vi "RunPWA_trigV2.vi"(4 "Software + buffering delay per pulse (s)":dbl=2e-06 format="%#_6e", 5 "trigger source":tag="/Dev1/PFI0", 6 "Analogue freq. (Hz)":dbl=5000.0 format="%0.2f", 7 "PW num. samples.":i32=400, 8 "PW freq. (Hz)":dbl=40.0) -> (0 "Drift of last pulse (mu. s)":dbl=-9.089951014118469e-10 format="%#_3g", 1 "Anl. / PW avg. jitter (mu.s)":dbl=212.9999999999574 format="%#_3g", 2 "Analogue data":dbl[][](array[numeric]) format="%.12f", 3 "I16 TOF (mu.s)":i16[](array[numeric])=[1380, 1279, 1463, 1254, 1163, 1317, 1629, 1097, 1100, 1774, 1172, 875, 1503, 1432, 1350, 1355, 1130, 951, 1434, 896, 1411, 1853, 1581, 1243, 1357, 886, 1545, 1268, 1475, 1942, 1228, 1498, 1306, 1554, 1663, 1181, 1453, 1038, 1198, 1321, 1316, 1534, 1316, 1839, 1620, 1542, 1789, 1374, 939, 1620, 1523, 1367, 1690, 1214, 1171, 1501, 955, 1457, 1429, 1619, 1347, 1398, 1041, 1123, 1263, 1106, 1795, 1222, 1683, 1818, 2362, 1402, 1544, 1060, 1109, 948, 1300, 1479, 1547, 1002, 1425, 1377, 2256, 1082, 1468, 2220, 1721, 1028, 1032, 1181, 1752, 1307, 1024, 1381, 1584, 1466, 1401, 902, 1473, 1422, 1798, 1715, 1444, 1316, 930, 1031, 1065, 1818, 1289, 2087, 1222, 1281, 1451, 1294, 1524, 1560, 1793, 1636, 1721, 1279, 1119, 1085, 1433, 1231, 1226, 1468, 1979, 1792, 2061, 1186, 1149, 1282, 1650, 1549, 1923, 1522, 1557, 1343, 1469, 1714, 1326, 1296, 1177, 1327, 1773, 1391, 1558, 1405, 1440, 1236, 1575, 1310, 1424, 1156, 1287, 731, 1458, 1393, 1493, 1441, 1196, 1605, 919, 1336, 1243, 1473, 1562, 1199, 1450, 1386, 1490, 1384, 1481, 1434, 1348, 1614, 1412, 1259, 2135, 1674, 1178, 1208, 1387, 1596, 1603, 1250, 1268, 1236, 1351, 1252, 1367, 1378, 1282, 1146, 1345, 1187, 1008, 1141, 1267, 1915, 1375, 1417, 1105, 1359, 1513, 1012, 1671, 1508, 1760, 1309, 1198, 1252, 1244, 1556, 1671, 1296, 1395, 1334, 1313, 1917, 1734, 1940, 1276, 1271, 1472, 1273, 981, 1430, 1391, 1038, 1236, 1167, 1419, 1935, 1188, 1658, 1317, 1217, 1663, 1432, 1498, 1494, 1620, 1528, 1200, 1603, 1200, 1514, 1288, 1327, 1644, 1311, 1573, 1033, 1669, 1022, 1624, 1999, 1993, 1489, 1519, 1483, 2032, 1397, 1345, 1706, 1229, 1299, 1063, 1269, 1192, 1609, 1377, 1299, 1538, 1347, 1231, 1262, 2060, 1816, 1442, 1713, 1096, 1593, 1807, 1549, 1242, 1353, 1506, 1533, 1551, 1097, 1770, 1588, 1253, 1313, 1345, 1658, 1527, 1551, 1780, 1001, 876, 1167, 1105, 1430, 1180, 1176, 1404, 785, 1377, 998, 1485, 1357, 952, 1304, 1477, 1138, 1303, 1281, 1376, 1603, 1495, 1690, 2050, 1558, 1238, 1430, 1341, 1126, 1070, 1743, 1649, 2205, 1470, 1632, 1677, 1210, 1669, 1968, 1267, 1394, 1582, 1865, 1256, 1582, 1356, 1535, 1791, 1637, 1226, 1787, 905, 1677, 1579, 876, 988, 1474, 1899, 1221, 1791, 1694, 1636, 1203, 1458, 1555, 1251, 1382, 954, 1185, 1240, 1264, 1228, 1298, 1885, 1489, 1702, 2401, 1725, 1110, 1190, 1572, 1369, 1223, 1131, 994, 1319, 1154, 1425, 1921, 1849, 1142, 1393, 1449, 1719, 1238, 1073, 1123, 1807, 1987])   [LabVIEW 2010]
uses:
  Kernel32.dll
  National Instruments/LabVIEW 2010/resource/objmgr/daqmx.rc
  PWAtasksGLOBAL.vi
  <vilib>/DAQmx/configure/timing.llb/DAQmx Timing (Sample Clock).vi
  <vilib>/DAQmx/configure/trigger.llb/DAQmx Start Trigger (Digital Edge).vi
  <vilib>/DAQmx/create/channels.llb/DAQmx Create Channel (DI-Digital Input).vi
  <vilib>/DAQmx/create/channels.llb/DAQmx Create Channel (DO-Digital Output).vi
  <vilib>/DAQmx/create/channels.llb/DAQmx Create Channel (AI-Voltage-Basic).vi
  <vilib>/DAQmx/read.llb/DAQmx Read (Analog 2D DBL NChan NSamp).vi
panel:
  in  "HW firing delay (s)":dbl=0.00085 format="%#_6e"
  in  "Save data?":bool
  in  "Path to save all data":path=path "C:/Documents and Settings/Aero Tunnel/Desktop/PWA vis, DAQmx and high res timer + HW/test.xls"
  in  "Analogue input channel(s)":tag="Dev1/ai0:2"
  out "PW compensated freq. (Hz)":dbl=40.003200256020484 format="%#.12g"
  in  "single shot mode for testing":bool
  out "Analogue Volts":cluster{dbl, dbl, "data":dbl[][]}(graph)={0.0, 0.0002, "data"=array3x50000[150000 elements]}
  out "PWA TOFs":cluster{"time":dbl[], i16[]}(graph)={"time"=array[400 elements], [1380, 1279, 1463, 1254, 1163, 1317, 1629, 1097, 1100, 1774, 1172, 875, 1503, 1432, 1350, 1355, 1130, 951, 1434, 896, 1411, 1853, 1581, 1243, 1357, 886, 1545, 1268, 1475, 1942, 1228, 1498, 1306, 1554, 1663, 1181, 1453, 1038, 1198, 1321, 1316, 1534, 1316, 1839, 1620, 1542, 1789, 1374, 939, 1620, 1523, 1367, 1690, 1214, 1171, 1501, 955, 1457, 1429, 1619, 1347, 1398, 1041, 1123, 1263, 1106, 1795, 1222, 1683, 1818, 2362, 1402, 1544, 1060, 1109, 948, 1300, 1479, 1547, 1002, 1425, 1377, 2256, 1082, 1468, 2220, 1721, 1028, 1032, 1181, 1752, 1307, 1024, 1381, 1584, 1466, 1401, 902, 1473, 1422, 1798, 1715, 1444, 1316, 930, 1031, 1065, 1818, 1289, 2087, 1222, 1281, 1451, 1294, 1524, 1560, 1793, 1636, 1721, 1279, 1119, 1085, 1433, 1231, 1226, 1468, 1979, 1792, 2061, 1186, 1149, 1282, 1650, 1549, 1923, 1522, 1557, 1343, 1469, 1714, 1326, 1296, 1177, 1327, 1773, 1391, 1558, 1405, 1440, 1236, 1575, 1310, 1424, 1156, 1287, 731, 1458, 1393, 1493, 1441, 1196, 1605, 919, 1336, 1243, 1473, 1562, 1199, 1450, 1386, 1490, 1384, 1481, 1434, 1348, 1614, 1412, 1259, 2135, 1674, 1178, 1208, 1387, 1596, 1603, 1250, 1268, 1236, 1351, 1252, 1367, 1378, 1282, 1146, 1345, 1187, 1008, 1141, 1267, 1915, 1375, 1417, 1105, 1359, 1513, 1012, 1671, 1508, 1760, 1309, 1198, 1252, 1244, 1556, 1671, 1296, 1395, 1334, 1313, 1917, 1734, 1940, 1276, 1271, 1472, 1273, 981, 1430, 1391, 1038, 1236, 1167, 1419, 1935, 1188, 1658, 1317, 1217, 1663, 1432, 1498, 1494, 1620, 1528, 1200, 1603, 1200, 1514, 1288, 1327, 1644, 1311, 1573, 1033, 1669, 1022, 1624, 1999, 1993, 1489, 1519, 1483, 2032, 1397, 1345, 1706, 1229, 1299, 1063, 1269, 1192, 1609, 1377, 1299, 1538, 1347, 1231, 1262, 2060, 1816, 1442, 1713, 1096, 1593, 1807, 1549, 1242, 1353, 1506, 1533, 1551, 1097, 1770, 1588, 1253, 1313, 1345, 1658, 1527, 1551, 1780, 1001, 876, 1167, 1105, 1430, 1180, 1176, 1404, 785, 1377, 998, 1485, 1357, 952, 1304, 1477, 1138, 1303, 1281, 1376, 1603, 1495, 1690, 2050, 1558, 1238, 1430, 1341, 1126, 1070, 1743, 1649, 2205, 1470, 1632, 1677, 1210, 1669, 1968, 1267, 1394, 1582, 1865, 1256, 1582, 1356, 1535, 1791, 1637, 1226, 1787, 905, 1677, 1579, 876, 988, 1474, 1899, 1221, 1791, 1694, 1636, 1203, 1458, 1555, 1251, 1382, 954, 1185, 1240, 1264, 1228, 1298, 1885, 1489, 1702, 2401, 1725, 1110, 1190, 1572, 1369, 1223, 1131, 994, 1319, 1154, 1425, 1921, 1849, 1142, 1393, 1449, 1719, 1238, 1073, 1123, 1807, 1987]}
  out "N samp. anl.":i32=50000
  out "Sampling time (s)":dbl=10.0
  out "TotalSampPerChanAcquired":dbl=50000.0
  out "AvailSampPerChan":u32
  out "CurrReadPos":dbl=50000.0
  out "Clock period (ns)":dbl=0.33336778133740486
  out "PW act. N. samps.":i32=400
  out "PW nominal dt (s)":dbl=0.025
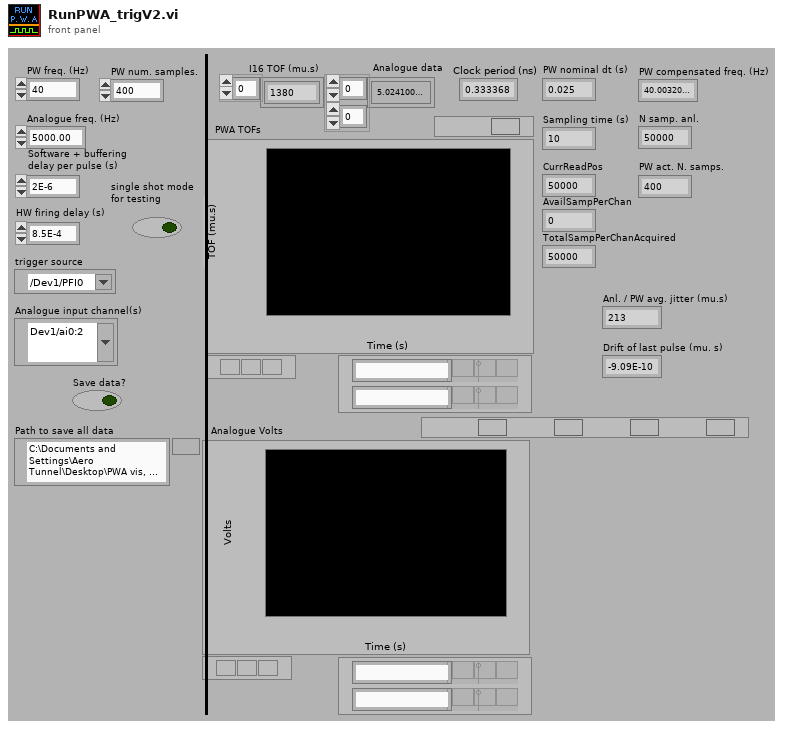
[diagram p1: front panel]
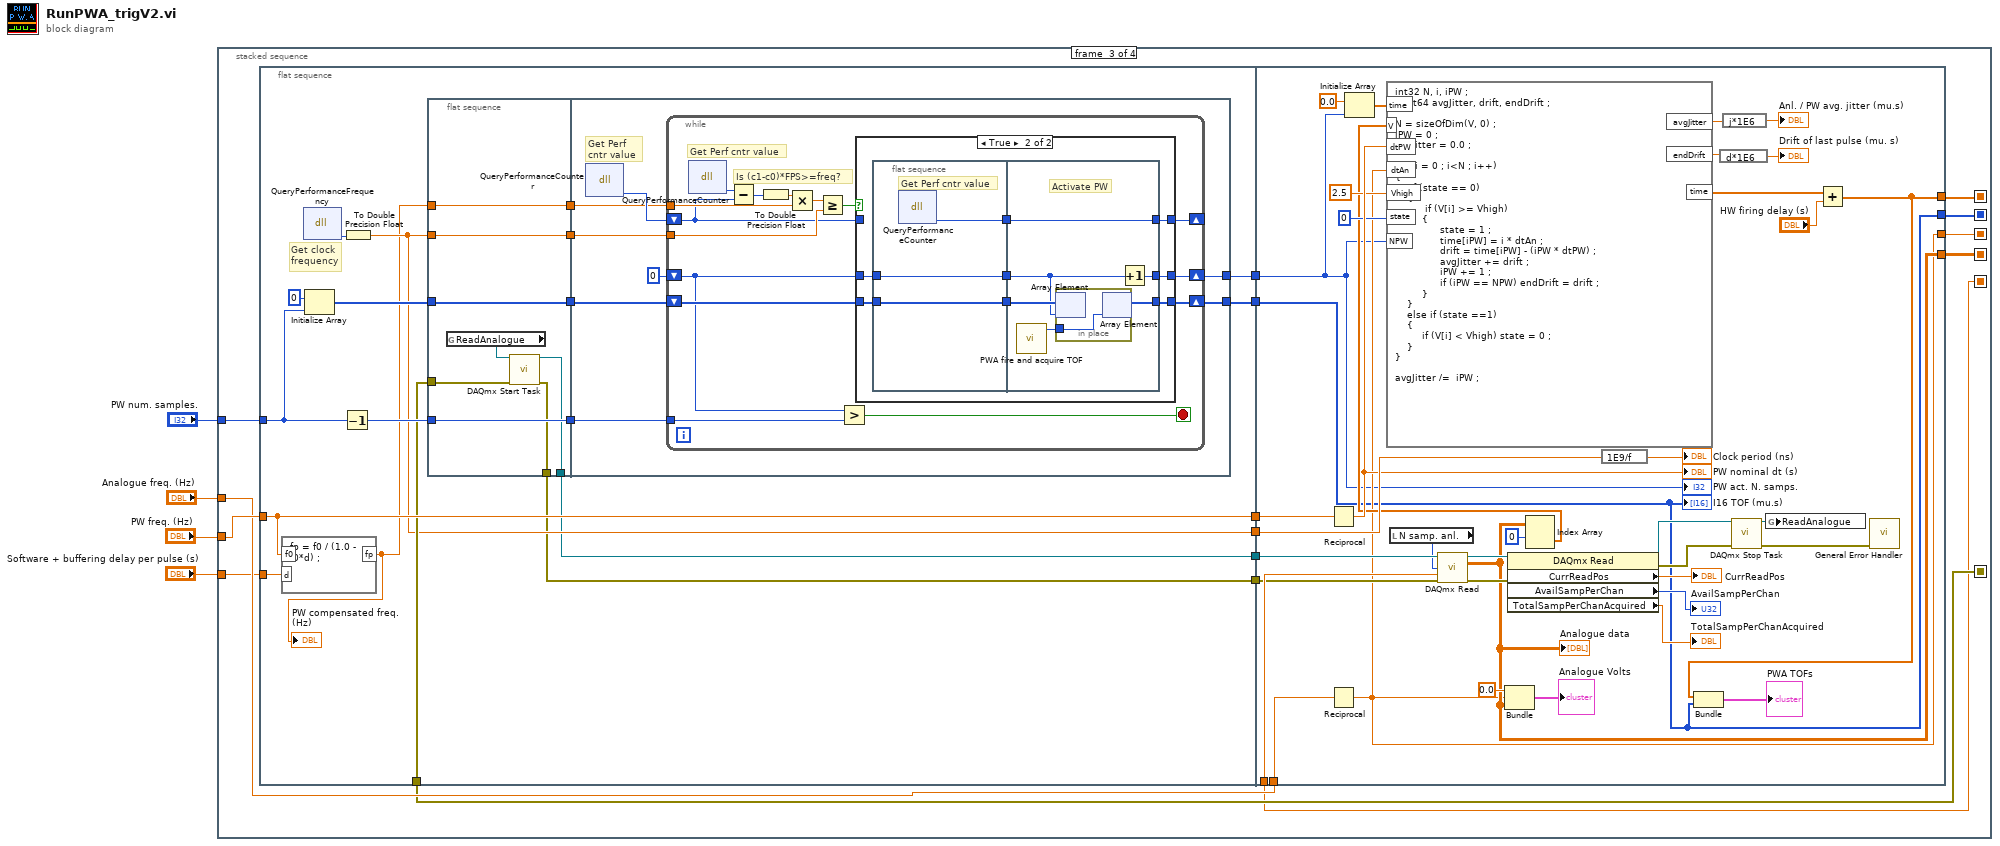
[diagram p0: block diagram]
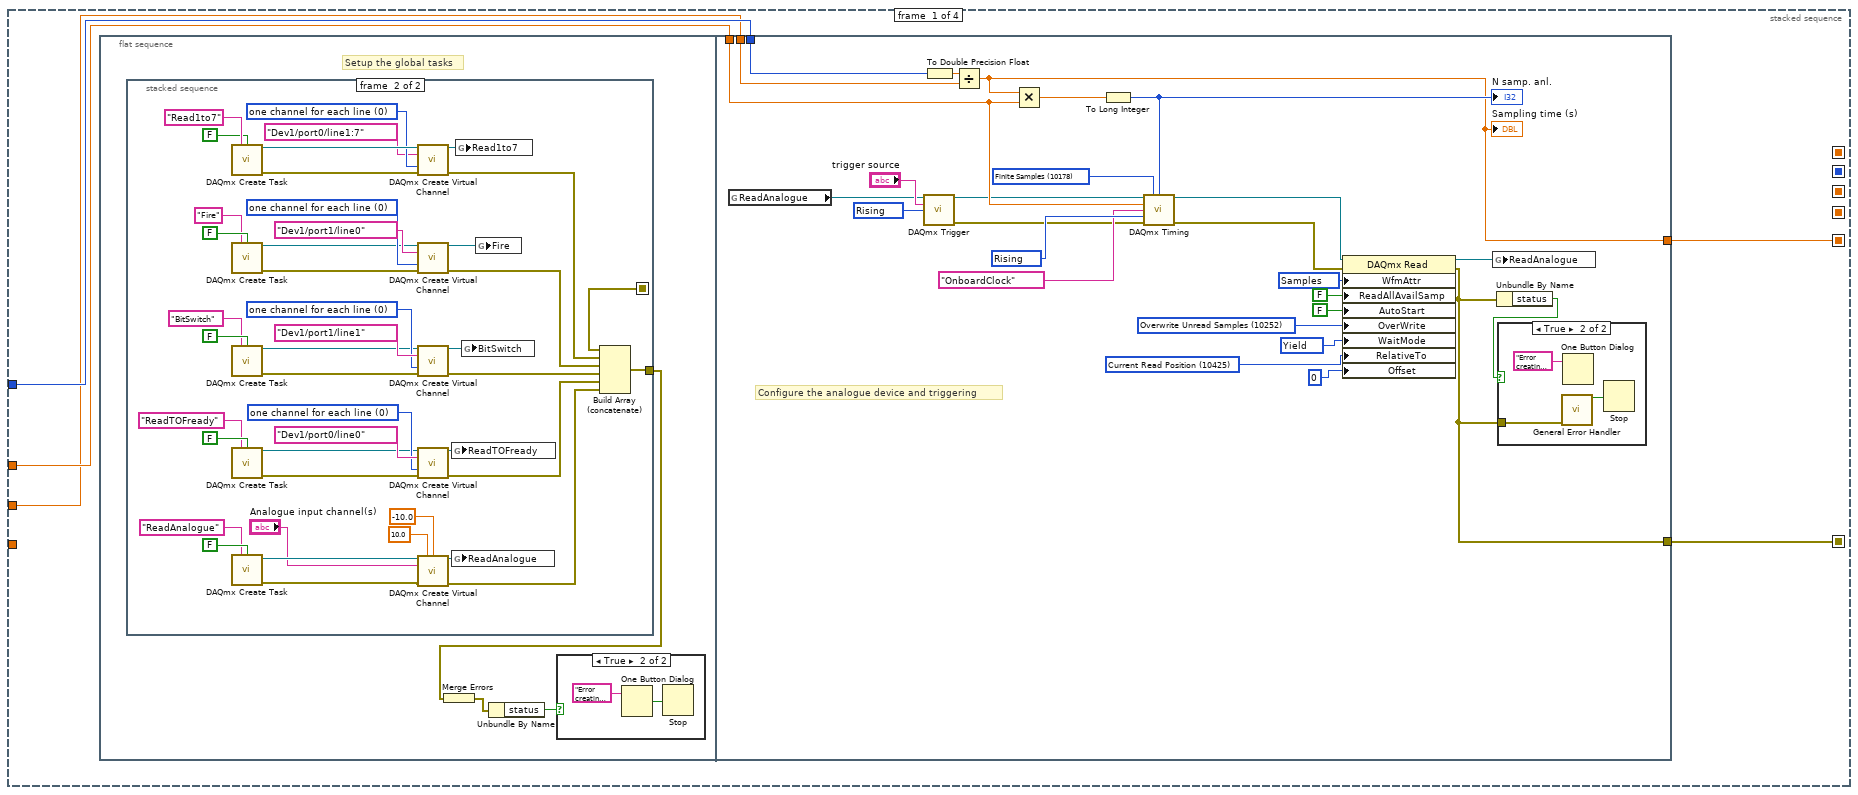
[diagram p2: hidden frame]
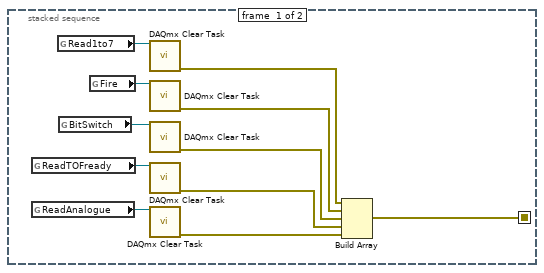
[diagram p3: hidden frame]
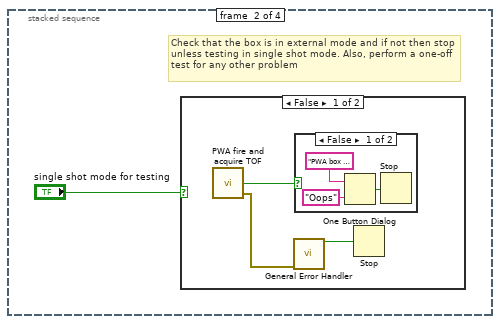
[diagram p6: hidden frame]
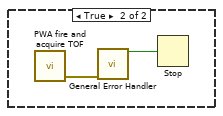
[diagram p8: hidden frame]
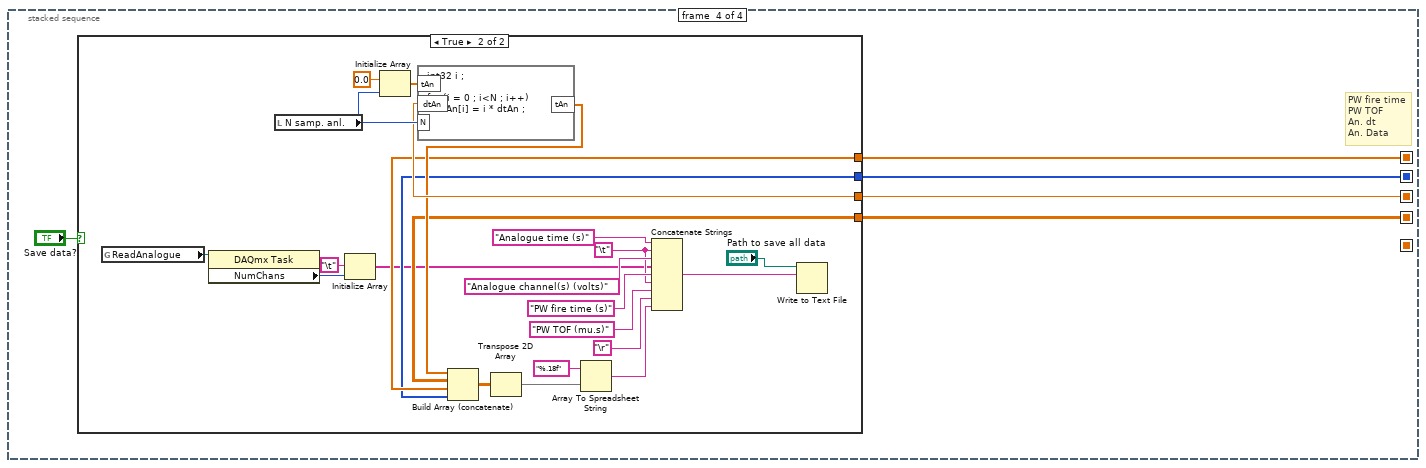
[diagram p10: hidden frame]
diagram:
  n1 = stacked-sequence {
    seq-local: [w8 _ _ _] -> [_ _ w115 _]
    seq-local: [w5 _ _ _] -> [_ _ w113 _]
    seq-local: [_ _ w111 _] -> [_ _ _ w234]
    seq-local: [_ _ w110 _] -> [_ _ _ w235]
    seq-local: [_ _ w109 _] -> [_ _ _ w236]
    seq-local: [_ _ w108 _] -> [_ _ _ w233]
    tunnel: "Analogue freq. (Hz)" -> [w9 _ w119 _]
    tunnel: "PW freq. (Hz)" -> [w6 _ w121 _]
    tunnel: "PW num. samples." -> [w7 _ w120 _]
    tunnel: "Software + buffering delay per pulse (s)" -> [_ _ w114 _]
    frame #0 {
      n2 = flat-sequence {
        tunnel: w9 -> [w81]
        tunnel: [w74] -> w8
        tunnel: w7 -> [w71]
        tunnel: w6 -> [w70]
        tunnel: [w69] -> w5
        frame #0 {
          # "Setup the global tasks"
          n3 = stacked-sequence {
            seq-local: [w13 _] -> [_ w30]
            tunnel: [_ w24] -> w11
            frame #0 {
              n4 = global read "PWAtasksGLOBAL.vi" "ReadTOFready"() -> (w20:refnum<k21>)
              n5 = global read "PWAtasksGLOBAL.vi" "ReadAnalogue"() -> (w19:refnum<k21>)
              n6 = global read "PWAtasksGLOBAL.vi" "Read1to7"() -> (w23:refnum<k21>)
              n7 = global read "PWAtasksGLOBAL.vi" "BitSwitch"() -> (w21:refnum<k21>)
              n8 = global read "PWAtasksGLOBAL.vi" "Fire"() -> (w22:refnum<k21>)
              n9 = call <vilib>:"DAQmx Clear Task.vi"("task in"=w23) -> ("error out"=w18:errorcluster)  [unwired: 14 in]
              n10 = call <vilib>:"DAQmx Clear Task.vi"("task in"=w22) -> ("error out"=w17:errorcluster)  [unwired: 14 in]
              n11 = call <vilib>:"DAQmx Clear Task.vi"("task in"=w21) -> ("error out"=w16:errorcluster)  [unwired: 14 in]
              n12 = call <vilib>:"DAQmx Clear Task.vi"("task in"=w20) -> ("error out"=w15:errorcluster)  [unwired: 14 in]
              n13 = call <vilib>:"DAQmx Clear Task.vi"("task in"=w19) -> ("error out"=w14:errorcluster)  [unwired: 14 in]
              n14 = Build Array(w18, w17, w16, w15, w14) -> (w13:errorcluster[])
            }
            frame #1 {
              w44 = 0 items=["one channel for each line", "one channel for all lines"] ("line grouping")
              w51 = 0 items=["one channel for each line", "one channel for all lines"] ("line grouping")
              w58 = 0 items=["one channel for each line", "one channel for all lines"] ("line grouping")
              w63 = 0 items=["one channel for each line", "one channel for all lines"] ("line grouping")
              n15 = call <vilib>:"DAQmx Create Task.vi"("new task name"="Read1to7", "auto cleanup"=FALSE) -> ("task out"=w64:refnum<k21>, "error out"=w60:errorcluster)  [unwired: 12 in]
              n16 = call <vilib>:"DAQmx Create Task.vi"("new task name"="Fire", "auto cleanup"=FALSE) -> ("task out"=w57:refnum<k21>, "error out"=w53:errorcluster)  [unwired: 12 in]
              n17 = call <vilib>:"DAQmx Create Task.vi"("new task name"="BitSwitch", "auto cleanup"=FALSE) -> ("task out"=w50:refnum<k21>, "error out"=w46:errorcluster)  [unwired: 12 in]
              n18 = call <vilib>:"DAQmx Create Task.vi"("new task name"="ReadTOFready", "auto cleanup"=FALSE) -> ("task out"=w43:refnum<k21>, "error out"=w39:errorcluster)  [unwired: 12 in]
              n19 = call <vilib>:"DAQmx Create Task.vi"("new task name"="ReadAnalogue", "auto cleanup"=FALSE) -> ("task out"=w38:refnum<k21>, "error out"=w34:errorcluster)  [unwired: 12 in]
              n20 = call-poly <vilib>:"DAQmx Create Virtual Channel.vi"("task in"=w64, "lines"=tag "Dev1/port0/line1:7", "line grouping"=w63, "error in"=w60) -> ("task out"=w61:refnum<k21>, "error out"=w29:errorcluster)  [unwired: 10 in]
              n21 = call-poly <vilib>:"DAQmx Create Virtual Channel.vi"("task in"=w57, "lines"=tag "Dev1/port1/line0", "line grouping"=w58, "error in"=w53) -> ("task out"=w54:refnum<k21>, "error out"=w28:errorcluster)  [unwired: 10 in]
              n22 = call-poly <vilib>:"DAQmx Create Virtual Channel.vi"("task in"=w50, "lines"=tag "Dev1/port1/line1", "line grouping"=w51, "error in"=w46) -> ("task out"=w47:refnum<k21>, "error out"=w27:errorcluster)  [unwired: 10 in]
              n23 = call-poly <vilib>:"DAQmx Create Virtual Channel.vi"("task in"=w43, "lines"=tag "Dev1/port0/line0", "line grouping"=w44, "error in"=w39) -> ("task out"=w40:refnum<k21>, "error out"=w26:errorcluster)  [unwired: 10 in]
              n24 = call-poly <vilib>:"DAQmx Create Virtual Channel.vi"("task in"=w38, "maximum value"=10.0, "minimum value"=-10.0, "physical channels"="Analogue input channel(s)", "error in"=w34) -> ("task out"=w35:refnum<k21>, "error out"=w25:errorcluster)  [unwired: 9 in]
              n25 = global write "PWAtasksGLOBAL.vi" "ReadTOFready"(w40) -> ()
              n26 = global write "PWAtasksGLOBAL.vi" "ReadAnalogue"(w35) -> ()
              n27 = global write "PWAtasksGLOBAL.vi" "Read1to7"(w61) -> ()
              n28 = global write "PWAtasksGLOBAL.vi" "BitSwitch"(w47) -> ()
              n29 = global write "PWAtasksGLOBAL.vi" "Fire"(w54) -> ()
              n30 = Build Array (concatenate)(w30, w29, w28, w27, w26, w25) -> (w24:errorcluster[])
            }
          }
          n31 = Merge Errors(w11) -> (w12:errorcluster)
          n32 = Unbundle By Name(w12) -> ("status"=w10:bool)
          n33 = case shown="True" w10 {
            frame False {
            }
            frame True {
              n34 = One Button Dialog(message="Error creating tasks, aborting") -> (true=w67:bool)  [unwired: 1 in]
              n35 = Stop(stop? (T)=w67) -> ()
            }
          }
        }
        frame #1 {
          w78 = 10280 items=["Rising"=10280, "Falling"=10171] ("edge")
          w87 = 10425 items=["First Sample"=10424, "Current Read Position"=10425, "Reference Trigger"=10426, "First Pretrigger Sample"=10427, "Most Recent Sample"=10428] ("RelativeTo")
          w88 = 12525 items=["Wait For Interrupt"=12523, "Poll"=12524, "Yield"=12525, "Sleep"=12547] ("WaitMode")
          w89 = 10252 items=["Overwrite Unread Samples"=10252, "Do Not Overwrite Unread Samples"=10159] ("OverWrite")
          w91 = 10287 items=["Samples"=10287, "Samples and Timing"=10140, "Samples, Timing, and Attributes"=10141] ("WfmAttr")
          w94 = 10280 items=["Rising"=10280, "Falling"=10171] ("active edge")
          w95 = 10178 items=["Finite Samples"=10178, "Continuous Samples"=10123, "Hardware Timed Single Point"=12522] ("sample mode")
          # "Configure the analogue device and triggering"
          n36 = global read "PWAtasksGLOBAL.vi" "ReadAnalogue"() -> (w73:refnum<k21>)
          n37 = call-poly <vilib>:"DAQmx Trigger.vi"("task/channels in"=w73, "source"="trigger source", "edge"=w78) -> ("task out"=w77:refnum<k21>, "error out"=w80:errorcluster)  [unwired: 11 in]
          n38 = To Double Precision Float(number=w71) -> (double precision float=w72:dbl)
          n39 = Divide(x=w72, y=w70) -> (x/y=w69:dbl)
          "Sampling time (s)" <- w69
          n40 = Multiply(x=w69, y=w81) -> (x*y=w83:dbl)
          n41 = To Long Integer(number=w83) -> (32bit integer=w82:i32)
          "N samp. anl." <- w82
          n42 = call-poly <vilib>:"DAQmx Timing.vi"("task/channels in"=w77, "sample mode"=w95, "samples per channel"=w82, "rate"=w81, "source"=tag "OnboardClock", "active edge"=w94, "error in"=w80) -> ("task out"=w76:refnum<k21>, "error out"=w85:errorcluster)  [unwired: 7 in]
          n43 = property class="DAQmx Read"(reference=w76, error in=w85, "WfmAttr"=w91, "ReadAllAvailSamp"=FALSE, "AutoStart"=FALSE, "OverWrite"=w89, "WaitMode"=w88, "RelativeTo"=w87, "Offset"=0) -> (reference out=w75:refnum<k21>, error out=w74:errorcluster)
          n44 = global write "PWAtasksGLOBAL.vi" "ReadAnalogue"(w75) -> ()
          n45 = Unbundle By Name(w74) -> ("status"=w84:bool)
          n46 = case shown="True" w84 {
            tunnel: w74 -> [_ w97]
            frame False {
            }
            frame True {
              n47 = call <vilib>:"General Error Handler.vi"("error in (no error)"=w97) -> ("error?"=w96:bool)  [unwired: 10 in, 4 out]
              n48 = One Button Dialog(message="Error creating tasks, aborting") -> ()  [unwired: 1 in, 1 out]
              n49 = Stop(stop? (T)=w96) -> ()
            }
          }
        }
      }
    }
    frame #1 {
      # "Check that the box is in external mode and if not then stop unless testing in single shot mode. Also, perform a one-off test for any other problem"
      n50 = case shown="False" "single shot mode for testing" {
        frame False {
          n51 = call "PWA fire and acquire TOF.vi"() -> ("Cumulative Error"=w100:errorcluster, "External mode"=w102:bool)  [unwired: 1 out]
          n52 = call <vilib>:"General Error Handler.vi"("error in (no error)"=w100) -> ("error?"=w101:bool)  [unwired: 10 in, 4 out]
          n53 = case shown="False" w102 {
            frame False {
              n54 = One Button Dialog(message="PWA box is not in external trigger mode!", button name ("OK")="Oops") -> (true=w103:bool)
              n55 = Stop(stop? (T)=w103) -> ()
            }
            frame True {
            }
          }
          n56 = Stop(stop? (T)=w101) -> ()
        }
        frame True {
          n57 = call "PWA fire and acquire TOF.vi"() -> ("Cumulative Error"=w107:errorcluster)  [unwired: 2 out]
          n58 = call <vilib>:"General Error Handler.vi"("error in (no error)"=w107) -> ("error?"=w106:bool)  [unwired: 10 in, 4 out]
          n59 = Stop(stop? (T)=w106) -> ()
        }
      }
    }
    frame #2 {
      n60 = flat-sequence {
        tunnel: [w132] -> w123
        tunnel: [w140] -> w122
        tunnel: [w139] -> w118
        tunnel: [w138] -> w117
        tunnel: [w124] -> w116
        tunnel: w115 -> [w137]
        tunnel: [w125] -> w112
        tunnel: w114 -> [w126]
        tunnel: w120 -> [w127]
        tunnel: w121 -> [w138]
        tunnel: w123 -> [w216]
        tunnel: w122 -> [w199]
        tunnel: w119 -> [w224]
        tunnel: w113 -> [w219]
        tunnel: w118 -> [w198]
        tunnel: w117 -> [w215]
        tunnel: w116 -> [w218]
        tunnel: w112 -> [w217]
        tunnel: [w195] -> w111
        tunnel: [w202] -> w110
        tunnel: [w201] -> w109
        tunnel: [w199] -> w108
        frame #0 {
          # "Get clock frequency"
          n61 = formula code="fp = f0 / (1.0 - f0*d) ;"("f0"=w138, "d"=w126) -> ("fp"=w130:dbl)
          "PW compensated freq. (Hz)" <- w130
          n62 = dll-call lib="Kernel32.dll" fn="QueryPerformanceFrequency"() -> ("Frequency"=w129:u64)  [unwired: 5 in, 2 out]
          n63 = Initialize Array(i16 0 ("Base 10 TOF (signed, \nmu.sec)"), w127) -> (w134:i16[])
          n64 = Decrement(x=w127) -> (x-1=w141:i32)
          n65 = To Double Precision Float(number=w129) -> (double precision float=w132:dbl)
          n66 = flat-sequence {
            tunnel: w137 -> [w147]
            tunnel: w141 -> [w149]
            tunnel: [w149] -> w136
            tunnel: [w146] -> w135
            tunnel: w134 -> [w146]
            tunnel: [w145] -> w133
            tunnel: w132 -> [w145]
            tunnel: [w144] -> w131
            tunnel: w130 -> [w144]
            tunnel: [w143] -> w125
            tunnel: [w142] -> w124
            tunnel: [w155] -> w140
            tunnel: [w153] -> w139
            tunnel: w136 -> [w156]
            tunnel: w135 -> [w152]
            tunnel: w133 -> [w151]
            tunnel: w131 -> [w150]
            frame #0 {
              n67 = global read "PWAtasksGLOBAL.vi" "ReadAnalogue"() -> (w148:refnum<k21>)
              n68 = call <vilib>:"DAQmx Start Task.vi"("task/channels in"=w148, "error in"=w147) -> ("task out"=w142:refnum<k21>, "error out"=w143:errorcluster)  [unwired: 12 in]
            }
            frame #1 {
              # "Get Perf cntr value"
              n69 = dll-call lib="Kernel32.dll" fn="QueryPerformanceCounter"() -> ("Counter value"=w154:u64)  [unwired: 5 in, 2 out]
              n70 = while {
                tunnel: w156 -> [w165]
                shift-right: [w172] -> _
                shift-left: w154 -> [w169]
                tunnel: w150 -> [w171]
                tunnel: w151 -> [w170]
                shift-right: [w168] -> w153
                shift-left: 0 ("Counter value") -> [w164]
                shift-right: [w167] -> w155
                shift-left: w152 -> [w166]
                stop <- w158 stop-if-true
                # "Is (c1-c0)*FPS>=freq?"
                # "Get Perf cntr value"
                n71 = dll-call lib="Kernel32.dll" fn="QueryPerformanceCounter"() -> ("Counter value"=w163:u64)  [unwired: 5 in, 2 out]
                n72 = Subtract(x=w163, y=w169) -> (x-y=w159:u64)
                n73 = To Double Precision Float(number=w159) -> (double precision float=w162:dbl)
                n74 = Multiply(x=w162, y=w171) -> (x*y=w160:dbl)
                n75 = Greater Or Equal?(x=w160, y=w170) -> (x >= y?=w161:bool)
                n76 = Greater?(x=w164, y=w165) -> (0:w158:bool)
                n77 = case shown="True" w161 {
                  tunnel: [w175 w183] -> w172
                  tunnel: w169 -> [w175 _]
                  tunnel: [w174 w182] -> w168
                  tunnel: w164 -> [w174 w181]
                  tunnel: [w173 w180] -> w167
                  tunnel: w166 -> [w173 w179]
                  frame False {
                    # "Continue looping\nuntil required time\nhas elapsed"
                  }
                  frame True {
                    n78 = flat-sequence {
                      tunnel: [w186] -> w178
                      tunnel: w181 -> [w185]
                      tunnel: [w185] -> w177
                      tunnel: w179 -> [w184]
                      tunnel: [w184] -> w176
                      tunnel: [w187] -> w183
                      tunnel: w178 -> [w187]
                      tunnel: [w192] -> w182
                      tunnel: w177 -> [w190]
                      tunnel: [w188] -> w180
                      tunnel: w176 -> [w191]
                      frame #0 {
                        # "Get Perf cntr value"
                        n79 = dll-call lib="Kernel32.dll" fn="QueryPerformanceCounter"() -> ("Counter value"=w186:u64)  [unwired: 5 in, 2 out]
                      }
                      frame #1 {
                        # "Activate PW"
                        n80 = call "PWA fire and acquire TOF.vi"() -> ("Base 10 TOF (signed, \nmu.sec) (I16)"=w189:i16)  [unwired: 2 out]
                        n81 = in-place {
                          in-place-border: w189 -> [w193]
                          n82 = in-place-array #1(w191, w190) -> ()  [unwired: 1 out]
                          n83 = in-place-array #1(w193) -> (w188:i16[])  [unwired: 1 out]
                        }
                        n84 = Increment(x=w190) -> (x+1=w192:i32)
                      }
                    }
                  }
                }
              }
            }
          }
        }
        frame #1 {
          n85 = Reciprocal(x=w215) -> (1/x=w214:dbl)
          "PW nominal dt (s)" <- w214
          n86 = Reciprocal(x=w224) -> (1/x=w201:dbl)
          n87 = Initialize Array(0.0 ("element"), w198) -> (w204:dbl[])
          n88 = local read "N samp. anl."() -> (w205:i32)
          n89 = call-poly <vilib>:"DAQmx Read.vi"("task/channels in"=w218, "number of samples per channel"=w205, "timeout"=w219, "error in"=w217) -> ("task out"=w230:refnum<k21>, "data"=w202:dbl[][], "error out"=w229:errorcluster)  [unwired: 9 in]
          "Analogue data" <- w202
          n90 = Bundle(0.0, w201, "data"=w202) -> (→"Analogue Volts":cluster{dbl, dbl, "data":dbl[][]})  [unwired: 1 in]
          n91 = property class="DAQmx Read"(reference=w230, error in=w229) -> (reference out=w221:refnum<k21>, error out=w220:errorcluster, "CurrReadPos"=→"CurrReadPos":dbl, "AvailSampPerChan"=→"AvailSampPerChan":u32, "TotalSampPerChanAcquired"=→"TotalSampPerChanAcquired":dbl)
          n92 = Index Array(array=w202, index (row)=0) -> (element=w206:dbl[])  [unwired: 1 in]
          n93 = formula code="int32 N, i, iPW ;\nfloat64 avgJitter, drift, endDrift ;\n\nN = sizeOfDim(V, 0) ;\niPW = 0 ;\navgJitter = 0.0 ;\n\nfor (i = 0 ; i<N ; i++)\n{\n     if (state == 0) \n    {\n          if (V[i] >= Vhigh)\n         {\n               state = 1 ;\n               time[iPW] = i * dtAn ;\n               drift = time[iPW] - (iPW * dtPW) ;\n               avgJitter += drift ;\n               iPW += 1 ;\n               if (iPW == NPW) endDrift = drift ;\n         }\n    }\n    else if (state ==1)\n    {\n         if (V[i] < Vhigh) state = 0 ;\n    }\n}\n\navgJitter /=  iPW ;"("dtPW"=w214, "dtAn"=w201, "V"=w206, "Vhigh"=2.5 ("input variable"), "state"=u8 0 ("Counter value"), "NPW"=w198, "time"=w204) -> ("avgJitter"=w210:dbl, "endDrift"=w209:dbl, "time"=w196:dbl[])
          n94 = expression code="1E9/f"(w216) -> (→"Clock period (ns)":dbl)
          n95 = expression code="d*1E6"(w209) -> (→"Drift of last pulse (mu. s)":dbl)
          n96 = expression code="j*1E6"(w210) -> (→"Anl. / PW avg. jitter (mu.s)":dbl)
          n97 = call <vilib>:"DAQmx Stop Task.vi"("task/channels in"=w221, "error in"=w220) -> ("task out"=w194:refnum<k21>, "error out"=w222:errorcluster)  [unwired: 12 in]
          n98 = global write "PWAtasksGLOBAL.vi" "ReadAnalogue"(w194) -> ()
          n99 = Add(x=w196, y="HW firing delay (s)") -> (x+y=w195:dbl[])
          n100 = Bundle(w195, w199) -> (→"PWA TOFs":cluster{dbl[], i16[]})  [unwired: 1 in]
          n101 = call <vilib>:"General Error Handler.vi"("error in (no error)"=w222) -> ()  [unwired: 10 in, 5 out]
          "PW act. N. samps." <- w198
          "I16 TOF (mu.s)" <- w199
        }
      }
    }
    frame #3 {
      # "PW fire time\nPW TOF\nAn. dt\nAn. Data"
      n102 = case shown="True" "Save data?" {
        tunnel: w236 -> [_ w257]
        tunnel: w235 -> [_ w251]
        tunnel: w234 -> [_ w250]
        tunnel: w233 -> [_ w249]
        frame False {
        }
        frame True {
          w241 = "\t"
          n103 = global read "PWAtasksGLOBAL.vi" "ReadAnalogue"() -> (w240:refnum<k21>)
          n104 = property class="DAQmx Task"(reference=w240) -> ("NumChans"=w239:u32)  [unwired: 1 in, 2 out]
          n105 = local read "N samp. anl."() -> (w258:i32)
          n106 = Initialize Array("\t", w239) -> (w237:string[])
          n107 = Initialize Array(0.0 ("element"), w258) -> (w259:dbl[])
          n108 = formula code="int32 i ;\n\nfor (i = 0 ; i<N ; i++)\n     tAn[i] = i * dtAn ;"("tAn"=w259, "dtAn"=w257, "N"=w258) -> ("tAn"=w252:dbl[])
          n109 = Build Array (concatenate)(w252, w251, w250, w249) -> (w248:dbl[][])
          n110 = Transpose 2D Array(2D array=w248) -> (transposed array=w245:dbl[][])
          n111 = Array To Spreadsheet String(array=w245, 3:"%.18f" ("format string")) -> (spreadsheet string=w246:string)  [unwired: 1 in]
          n112 = Concatenate Strings("Analogue time (s)" ("initial string"), w241, "Analogue channel(s) (volts)" ("initial string"), w237, "PW fire time (s)" ("initial string"), w241, "PW TOF (mu.s)" ("initial string"), "\r", w246) -> (w243:string)
          n113 = Write to Text File(file (use dialog)="Path to save all data", text=w243) -> ()  [unwired: 2 in, 3 out]
        }
      }
    }
  }
